vi "povezivanje_mreynih.vi"() -> ()   [LabVIEW 2014]
panel:
  out "error out":errorcluster
  in  "error in (no error)":errorcluster
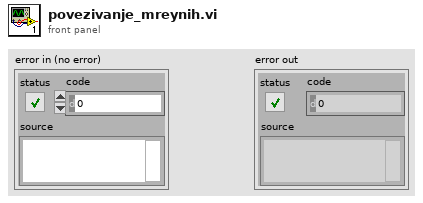
[diagram p1: front panel]
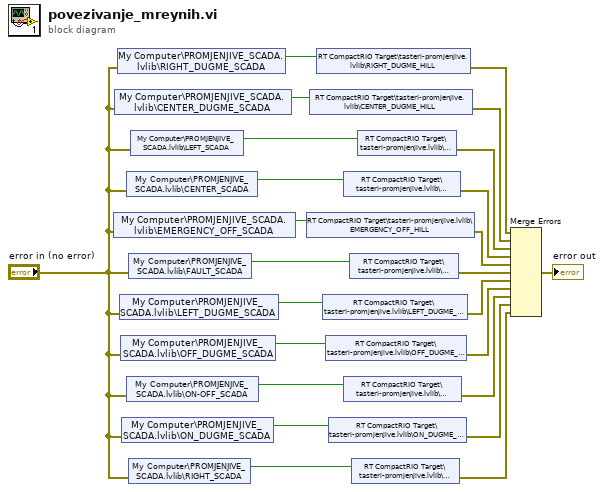
[diagram p0: block diagram]
diagram:
  n1 = shared-variable "My Computer\\PROMJENJIVE_SCADA.lvlib\\EMERGENCY_OFF_SCADA"(error in="error in (no error)") -> (w19:bool)  [unwired: 1 out]
  n2 = shared-variable "My Computer\\PROMJENJIVE_SCADA.lvlib\\CENTER_DUGME_SCADA"(error in="error in (no error)") -> (w22:bool)  [unwired: 1 out]
  n3 = shared-variable "My Computer\\PROMJENJIVE_SCADA.lvlib\\RIGHT_DUGME_SCADA"(error in="error in (no error)") -> (w23:bool)  [unwired: 1 out]
  n4 = shared-variable "My Computer\\PROMJENJIVE_SCADA.lvlib\\LEFT_DUGME_SCADA"(error in="error in (no error)") -> (w24:bool)  [unwired: 1 out]
  n5 = shared-variable "My Computer\\PROMJENJIVE_SCADA.lvlib\\OFF_DUGME_SCADA"(error in="error in (no error)") -> (w15:bool)  [unwired: 1 out]
  n6 = shared-variable "My Computer\\PROMJENJIVE_SCADA.lvlib\\ON_DUGME_SCADA"(error in="error in (no error)") -> (w14:bool)  [unwired: 1 out]
  n7 = shared-variable "RT CompactRIO Target\\tasteri-promjenjive.lvlib\\EMERGENCY_OFF_HILL"(w19) -> (error out=w8:errorcluster)  [unwired: 1 in]
  n8 = shared-variable "RT CompactRIO Target\\tasteri-promjenjive.lvlib\\CENTER_DUGME_HILL"(w22) -> (error out=w11:errorcluster)  [unwired: 1 in]
  n9 = shared-variable "RT CompactRIO Target\\tasteri-promjenjive.lvlib\\RIGHT_DUGME_HILL"(w23) -> (error out=w12:errorcluster)  [unwired: 1 in]
  n10 = shared-variable "RT CompactRIO Target\\tasteri-promjenjive.lvlib\\LEFT_DUGME_HILL"(w24) -> (error out=w6:errorcluster)  [unwired: 1 in]
  n11 = shared-variable "RT CompactRIO Target\\tasteri-promjenjive.lvlib\\OFF_DUGME_HILL"(w15) -> (error out=w5:errorcluster)  [unwired: 1 in]
  n12 = shared-variable "RT CompactRIO Target\\tasteri-promjenjive.lvlib\\ON_DUGME_HILL"(w14) -> (error out=w3:errorcluster)  [unwired: 1 in]
  n13 = shared-variable "RT CompactRIO Target\\tasteri-promjenjive.lvlib\\CENTER_HILL"() -> (w20:bool, error out=w9:errorcluster)  [unwired: 1 in]
  n14 = shared-variable "My Computer\\PROMJENJIVE_SCADA.lvlib\\CENTER_SCADA"(w20, error in="error in (no error)") -> ()  [unwired: 1 out]
  n15 = shared-variable "RT CompactRIO Target\\tasteri-promjenjive.lvlib\\ON-OFF_HILL"() -> (w17:bool, error out=w4:errorcluster)  [unwired: 1 in]
  n16 = shared-variable "My Computer\\PROMJENJIVE_SCADA.lvlib\\ON-OFF_SCADA"(w17, error in="error in (no error)") -> ()  [unwired: 1 out]
  n17 = shared-variable "RT CompactRIO Target\\tasteri-promjenjive.lvlib\\FAULT_HILL"() -> (w18:bool, error out=w7:errorcluster)  [unwired: 1 in]
  n18 = shared-variable "My Computer\\PROMJENJIVE_SCADA.lvlib\\FAULT_SCADA"(w18, error in="error in (no error)") -> ()  [unwired: 1 out]
  n19 = shared-variable "RT CompactRIO Target\\tasteri-promjenjive.lvlib\\RIGHT_HILL"() -> (w16:bool, error out=w2:errorcluster)  [unwired: 1 in]
  n20 = shared-variable "My Computer\\PROMJENJIVE_SCADA.lvlib\\RIGHT_SCADA"(w16, error in="error in (no error)") -> ()  [unwired: 1 out]
  n21 = shared-variable "RT CompactRIO Target\\tasteri-promjenjive.lvlib\\LEFT_HILL"() -> (w21:bool, error out=w10:errorcluster)  [unwired: 1 in]
  n22 = shared-variable "My Computer\\PROMJENJIVE_SCADA.lvlib\\LEFT_SCADA"(w21, error in="error in (no error)") -> ()  [unwired: 1 out]
  n23 = Merge Errors(w12, w11, w10, w9, w8, w7, w6, w5, w4, w3, w2) -> (→"error out":errorcluster)
